vi "Return Msg.vi"(8 "error in (no error)":errorcluster, 11 "Delete Control_Behavior.lvclass":refnum<class "Delete Control_Behavior.lvclass">) -> (0 "error out":errorcluster, 2 "Console Reply.lvclass":refnum<class "Console Reply.lvclass">, 3 "Panel Behavior(Class)":refnum<class "Panel Behavior.lvclass">)   [LabVIEW 2015, in "Delete Control_Behavior.lvclass"]
uses:
  Delete Control_Behavior.lvclass
  _Depences/Panel API/Panel Request/Panle Requeset Behavior/Panel Behavior.lvclass
  _Depences/Panel API/Console Reply/Console Reply/Console Reply.lvclass
  Console Reply Delete Control Result/Console Reply Delete Control.lvclass
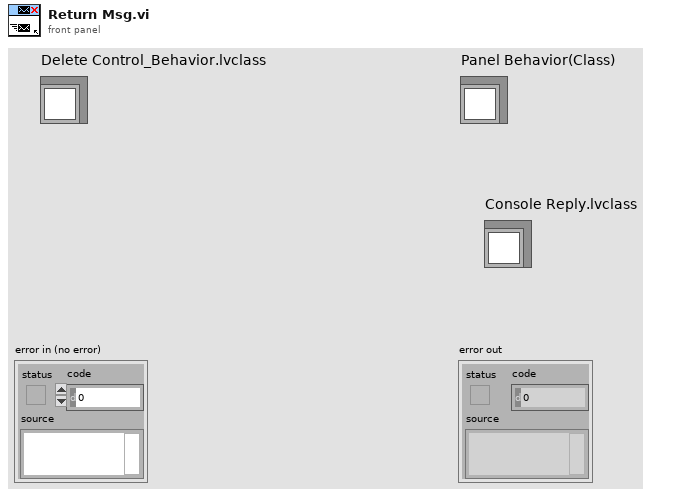
[diagram p1: front panel]
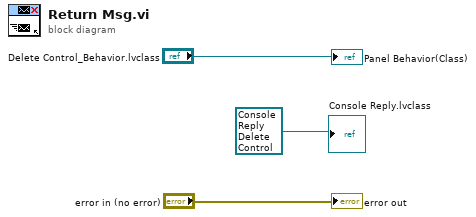
[diagram p0: block diagram]
diagram:
  "error out" <- "error in (no error)"
  "Panel Behavior(Class)" <- "Delete Control_Behavior.lvclass"
  "Console Reply.lvclass" <- refnum<class "Console Reply Delete Control.lvclass"> refnum ("Console Reply Delete Control.lvclass")
